vi "getStatusString.vi"(8 "error in (no error)":errorcluster, 11 "Status in":refnum<class "Status.lvclass">) -> (0 "error out":errorcluster, 2 "Status String":string, 3 "Status out":refnum<class "Status.lvclass">)   [LabVIEW 2017, in "Message Interface.lvlib" / "Status.lvclass"]
uses:
  Status.lvclass
  Status.lvclass/Status.ctl
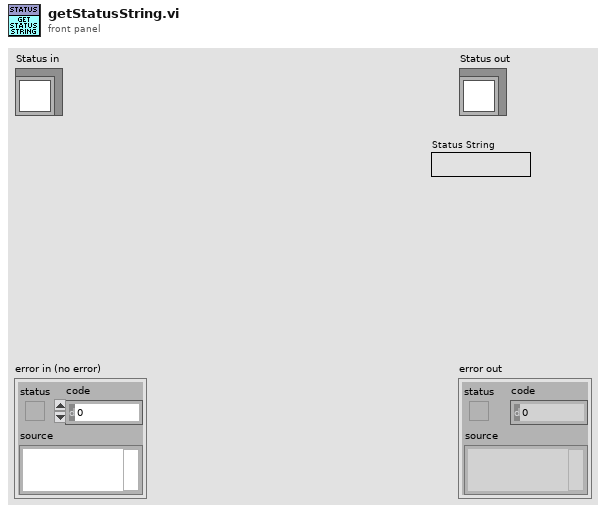
[diagram p1: front panel]
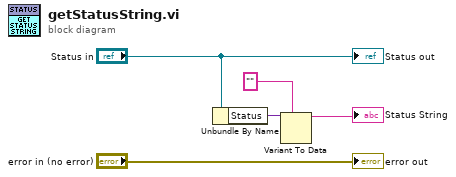
[diagram p0: block diagram]
diagram:
  n1 = Unbundle By Name("Status in") -> ("Status"=w3:variant)
  n2 = Variant To Data(type="", Variant=w3) -> (data=→"Status String":string)  [unwired: 1 in, 1 out]
  "error out" <- "error in (no error)"
  "Status out" <- "Status in"
